vi "Glocal Error Stop.vi"(6 "Force Stop":bool, 7 "Clear":bool, 10 "Error In":errorcluster) -> (2 "Output":bool)   [LabVIEW 2015]
panel:
  out "Error Out":errorcluster
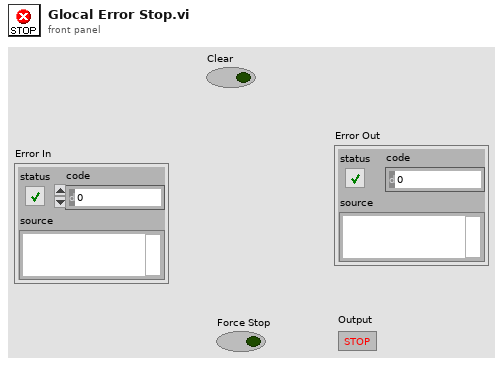
[diagram p1: front panel]
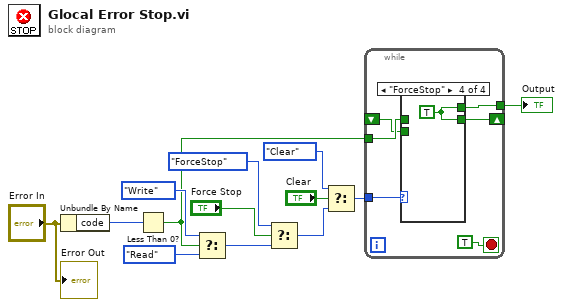
[diagram p0: block diagram]
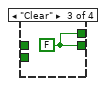
[diagram p4: hidden frame]
diagram:
  n1 = Unbundle By Name("Error In") -> ("code"=w12:i32)
  n2 = Less Than 0?(x=w12) -> (x < 0?=w10:bool)
  n3 = Select(t=enum16{"Write", "Read", "Clear", "ForceStop"}."Write" ("Enum"), s=w10, f=enum16{"Write", "Read", "Clear", "ForceStop"}."Read" ("Enum")) -> (s? t:f=w2:enum16{"Write", "Read", "Clear", "ForceStop"})
  n4 = Select(t=enum16{"Write", "Read", "Clear", "ForceStop"}."ForceStop" ("Enum"), s="Force Stop", f=w2) -> (s? t:f=w1:enum16{"Write", "Read", "Clear", "ForceStop"})
  n5 = Select(t=enum16{"Write", "Read", "Clear", "ForceStop"}."Clear" ("Enum"), s="Clear", f=w1) -> (s? t:f=w7:enum16{"Write", "Read", "Clear", "ForceStop"})
  n6 = while {
    tunnel: w10 -> [w19]
    shift-right: [w18] -> _
    shift-left: _ -> [w16]
    tunnel: [w17] -> w13
    tunnel: w7 -> [w14]
    stop <- TRUE stop-if-true
    n7 = case shown="\"ForceStop\"" w14 {
      tunnel: w19 -> [w20 _ _ _]
      tunnel: [w20 w21 w22 w23] -> w18
      tunnel: [w20 w21 w22 w23] -> w17
      tunnel: w16 -> [_ w21 _ _]
      frame "Write" {
      }
      frame "Read", Default {
      }
      frame "Clear" {
        w22 = FALSE
      }
      frame "ForceStop" {
        w23 = TRUE
      }
    }
  }
  "Output" <- w13
  "Error Out" <- "Error In"
